vi "UI.Sequence.SetRowWidths.vi"(8 "error in (no error)":errorcluster, 10 "CellSize":T1[](array[typedef]), 11 "UI.SequenceRef":refnum<vi>) -> (0 "error out":errorcluster, 3 "UI.SequenceRef":refnum<vi>)   [LabVIEW 2015, in "Simple Sequence Tools - Shared.lvlib"]
uses:
  Simple Sequence Tools - Shared.lvlib
  <vilib>/Utility/miscctls.llb/LVBoundsTypeDef.ctl
  <vilib>/Utility/miscctls.llb/LVRowAndColumnTypeDef.ctl
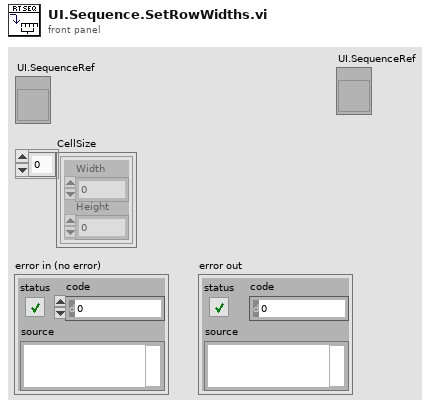
[diagram p1: front panel]
types:
  T1 = typedef "LVBoundsTypeDef.ctl" = cluster{"Width":u32, "Height":u32}
  T2 = typedef "LVRowAndColumnTypeDef.ctl" = cluster{"Row":i32, "Column":i32}
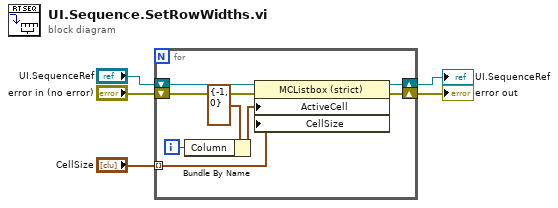
[diagram p0: block diagram]
diagram:
  n1 = for {
    shift-right: [w10] -> w1
    shift-left: "UI.SequenceRef" -> [w11]
    shift-right: [w12] -> w4
    shift-left: "error in (no error)" -> [w13]
    tunnel: "CellSize" -> [w6] mode=indexing
    i -> [w9]
    n2 = Bundle By Name(cluster=T2 {"Row"=-1, "Column"=0} ("Active Cell:Active Cell"), "Column"=w9) -> (w7:T2)
    n3 = property class="MCListbox (strict)"(reference=w11, error in=w13, "ActiveCell"=w7, "CellSize"=w6) -> (reference out=w10:refnum<vi>, error out=w12:errorcluster)
  }
  "error out" <- w4
  "UI.SequenceRef" <- w1
